vi "Test Debug Decorator.vi"() -> ()   [LabVIEW 2019]
uses:
  Attribute.Debug/DebugBehavior.ctl
  <vilib>/JKI/JKI SMO/SMO/SMO.lvclass
  SMO Debug.lvlib
  Attribute.Debug/Attribute.Debug.lvclass
panel:
  in  "Behavior":T1
  out "Behavior":T1
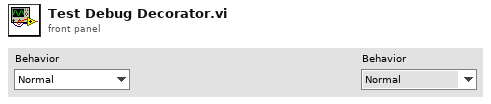
[diagram p1: front panel]
types:
  T1 = typedef "SMO Debug.lvlib/Attribute.Debug.lvclass/DebugBehavior.ctl" = enum16{"Normal", "Debug"}
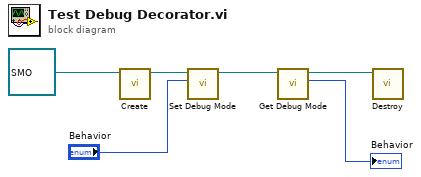
[diagram p0: block diagram]
diagram:
  n1 = call <vilib>:"Create.vi"("SMO"=refnum<class "SMO.lvclass"> refnum) -> ("SMO out"=w3:refnum<class "SMO.lvclass">)  [unwired: 8 in, 2 out]
  n2 = call "Set Debug Mode.vi"("Behavior"="Behavior", "SMO"=w3) -> ("SMO out"=w2:refnum<class "SMO.lvclass">)  [unwired: 8 in, 1 out]
  n3 = call "Get Debug Mode.vi"("SMO"=w2) -> ("Behavior"=→"Behavior":T1, "SMO out"=w5:refnum<class "SMO.lvclass">)  [unwired: 8 in, 1 out]
  n4 = call <vilib>:"Destroy.vi"("SMO"=w5) -> ()  [unwired: 10 in, 1 out]
